vi "assignment_one.vi"() -> ()   [LabVIEW 2015]
panel:
  in  "Reset":bool
  in  "Grab Soda (Reset)":bool
  out "Change Returned":dbl
  out "Change Deposited":dbl
  out "Dispense Soda":bool
  in  "Quarter":bool
  in  "Dime":bool
  in  "Nickel":bool
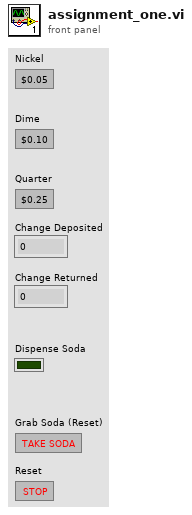
[diagram p1: front panel]
types:
  T1 = enum16{"Start", "5 cents", "10 cents", "15 cents", "20 cents", "25 cents", "30 cents", "35 cents", "40 cents", "45 cents"}
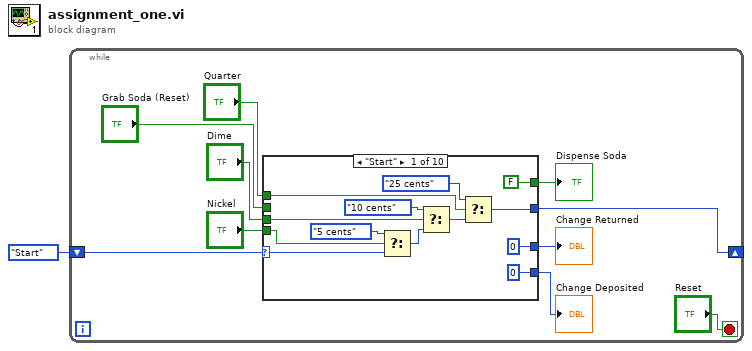
[diagram p0: block diagram]
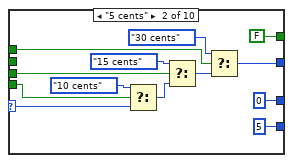
[diagram p2: hidden frame]
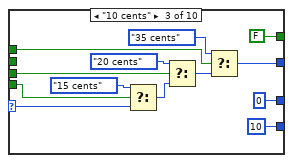
[diagram p3: hidden frame]
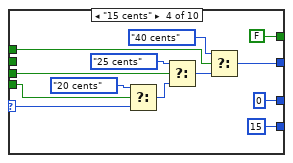
[diagram p4: hidden frame]
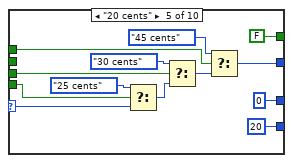
[diagram p5: hidden frame]
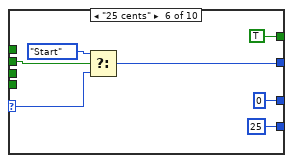
[diagram p6: hidden frame]
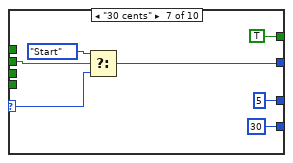
[diagram p7: hidden frame]
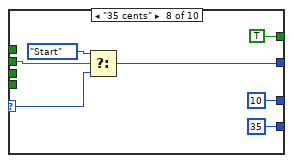
[diagram p8: hidden frame]
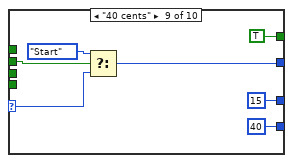
[diagram p9: hidden frame]
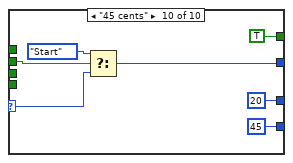
[diagram p10: hidden frame]
diagram:
  n1 = while {
    shift-right: [w4] -> _
    shift-left: T1."Start" -> [w11]
    stop <- "Reset" stop-if-true
    n2 = case shown="\"Start\"" w11 {
      selector: w11 -> [w19 w29 w38 w51 w64 w79 w88 w91 w101 w105]
      tunnel: "Nickel" -> [w21 w30 w39 w52 w65 _ _ _ _ _]
      tunnel: "Dime" -> [w17 w31 w40 w53 w66 _ _ _ _ _]
      tunnel: "Quarter" -> [w14 w32 w41 w54 w67 _ _ _ _ _]
      tunnel: [0 5 10 15 20 25 30 35 40 45] -> w7
      tunnel: [0 0 0 0 0 0 5 10 15 20] -> w6
      tunnel: [FALSE FALSE FALSE FALSE FALSE TRUE TRUE TRUE TRUE TRUE] -> w5
      tunnel: [w12 w28 w42 w55 w68 w77 w87 w96 w103 w110] -> w4
      tunnel: "Grab Soda (Reset)" -> [_ _ _ _ _ w80 w89 w92 w102 w106]
      frame "Start" {
        n3 = Select(t=T1."5 cents", s=w21, f=w19) -> (s? t:f=w18:T1)
        n4 = Select(t=T1."10 cents", s=w17, f=w18) -> (s? t:f=w13:T1)
        n5 = Select(t=T1."25 cents", s=w14, f=w13) -> (s? t:f=w12:T1)
      }
      frame "5 cents" {
        n6 = Select(t=T1."10 cents", s=w30, f=w29) -> (s? t:f=w36:T1)
        n7 = Select(t=T1."15 cents", s=w31, f=w36) -> (s? t:f=w33:T1)
        n8 = Select(t=T1."30 cents", s=w32, f=w33) -> (s? t:f=w28:T1)
      }
      frame "10 cents" {
        n9 = Select(t=T1."15 cents", s=w39, f=w38) -> (s? t:f=w47:T1)
        n10 = Select(t=T1."20 cents", s=w40, f=w47) -> (s? t:f=w50:T1)
        n11 = Select(t=T1."35 cents", s=w41, f=w50) -> (s? t:f=w42:T1)
      }
      frame "15 cents" {
        n12 = Select(t=T1."20 cents", s=w52, f=w51) -> (s? t:f=w60:T1)
        n13 = Select(t=T1."25 cents", s=w53, f=w60) -> (s? t:f=w63:T1)
        n14 = Select(t=T1."40 cents", s=w54, f=w63) -> (s? t:f=w55:T1)
      }
      frame "20 cents" {
        n15 = Select(t=T1."25 cents", s=w65, f=w64) -> (s? t:f=w75:T1)
        n16 = Select(t=T1."30 cents", s=w66, f=w75) -> (s? t:f=w72:T1)
        n17 = Select(t=T1."45 cents", s=w67, f=w72) -> (s? t:f=w68:T1)
      }
      frame "25 cents" {
        n18 = Select(t=T1."Start", s=w80, f=w79) -> (s? t:f=w77:T1)
      }
      frame "30 cents" {
        n19 = Select(t=T1."Start", s=w89, f=w88) -> (s? t:f=w87:T1)
      }
      frame "35 cents" {
        n20 = Select(t=T1."Start", s=w92, f=w91) -> (s? t:f=w96:T1)
      }
      frame "40 cents" {
        n21 = Select(t=T1."Start", s=w102, f=w101) -> (s? t:f=w103:T1)
      }
      frame "45 cents" {
        n22 = Select(t=T1."Start", s=w106, f=w105) -> (s? t:f=w110:T1)
      }
    }
    "Dispense Soda" <- w5
    "Change Deposited" <- w7
    "Change Returned" <- w6
  }
